vi "IncludeProject_IgnoreItemsInPrivateScope_WhitelistNotContainsFile.vi"(10 "expected_file":path) -> (0 "error out":errorcluster)   [LabVIEW 2017, in "Whitelist.Tests.lvlib"]
uses:
  Whitelist.Tests.lvlib
  Whitelist/Whitelist.lvclass
  Assertion/Assertion.lvlib
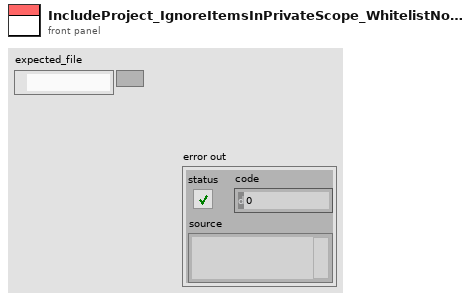
[diagram p1: front panel]
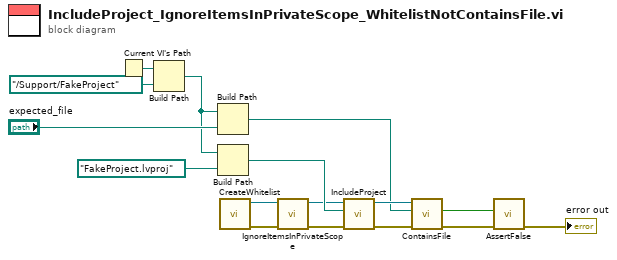
[diagram p0: block diagram]
diagram:
  n1 = Current VI's Path() -> (path=w9:path)
  n2 = Build Path(base path=w9, name or relative path=path "../Support/FakeProject" ("base path")) -> (appended path=w7:path)
  n3 = Build Path(base path=w7, name or relative path="expected_file") -> (appended path=w4:path)
  n4 = Build Path(base path=w7, name or relative path=path "FakeProject.lvproj") -> (appended path=w5:path)
  n5 = call "CreateWhitelist.vi"() -> ("error out"=w13:errorcluster, "Whitelist out"=w1:refnum<class "Whitelist.lvclass">)  [unwired: 10 in]
  n6 = call "IgnoreItemsInPrivateScope.vi"("error in (no error)"=w13, "Whitelist in"=w1) -> ("error out"=w3:errorcluster, "Whitelist out"=w2:refnum<class "Whitelist.lvclass">)  [unwired: 8 in]
  n7 = call "IncludeProject.vi"("error in (no error)"=w3, "Path"=w5, "Whitelist in"=w2) -> ("error out"=w12:errorcluster, "Whitelist out"=w11:refnum<class "Whitelist.lvclass">)  [unwired: 7 in]
  n8 = call "ContainsFile.vi"("error in (no error)"=w12, "Path"=w4, "Whitelist in"=w11) -> ("error out"=w16:errorcluster, "Is Whitelisted?"=w15:bool)  [unwired: 6 in, 1 out]
  n9 = call "AssertFalse.vi"("error in (no error)"=w16, "Condition"=w15) -> ("error out"=→"error out":errorcluster)  [unwired: 9 in]
